vi "Strings and Formats.vi"(0 "TTLControl in":refnum<class "TTLWaterController.lvclass">, 11 "error in (no error)":errorcluster) -> (4 "TTLControl out":refnum<class "TTLWaterController.lvclass">, 8 "Strings[] and Formats[]":cluster{"Strings":string[], "Formats":string[]}, 15 "error out":errorcluster)   [LabVIEW 2020, in "TTLWaterController.lvclass"]
uses:
  TTLWaterController.lvclass
  Base Class/TTLController.lvclass
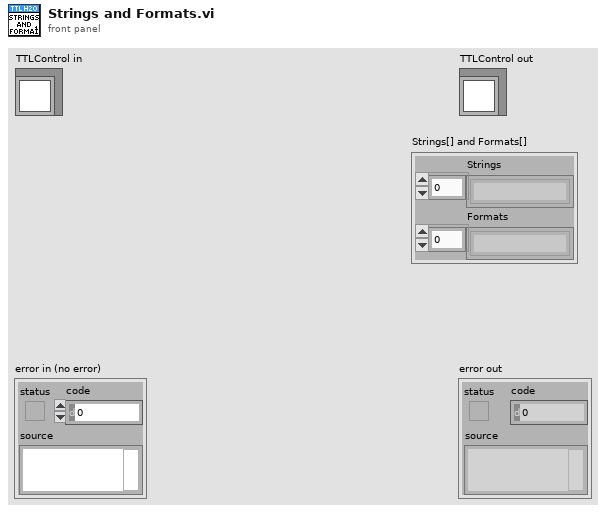
[diagram p1: front panel]
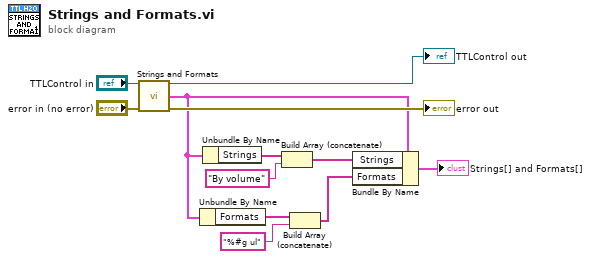
[diagram p0: block diagram]
diagram:
  n1 = call-parent "Strings and Formats.vi"("TTLControl in"="TTLControl in", "error in (no error)"="error in (no error)") -> ("TTLControl out"=→"TTLControl out":refnum<class "TTLWaterController.lvclass">, "Strings[] and Formats[]"=w4:cluster{"Strings":string[], "Formats":string[]}, "error out"=→"error out":errorcluster)  [unwired: 11 in]
  n2 = Unbundle By Name(w4) -> ("Formats"=w6:string[])
  n3 = Unbundle By Name(w4) -> ("Strings"=w8:string[])
  n4 = Build Array (concatenate)(w8, "By volume" ("String")) -> (w3:string[])
  n5 = Build Array (concatenate)(w6, "%#g ul" ("String")) -> (w2:string[])
  n6 = Bundle By Name(cluster=w4, "Strings"=w3, "Formats"=w2) -> (→"Strings[] and Formats[]":cluster{"Strings":string[], "Formats":string[]})
